vi "test number array to sgl array.vi"(10 "send values":string[](array[string])=["2", "19", "924", "0"]) -> (2 "sgl array":dbl[](array[numeric]))   [LabVIEW 2020]
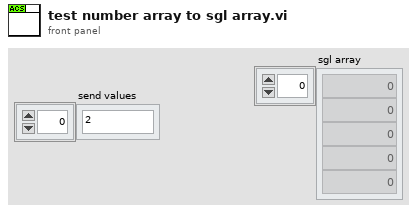
[diagram p1: front panel]
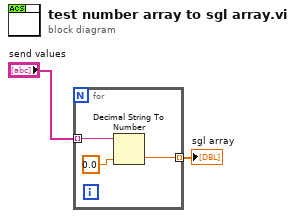
[diagram p0: block diagram]
diagram:
  n1 = for {
    tunnel: "send values" -> [w5] mode=indexing
    tunnel: [w3] -> w1 mode=indexing
    n2 = Decimal String To Number(string=w5, default (0L)=0.0) -> (number=w3:dbl)  [unwired: 1 in, 1 out]
  }
  "sgl array" <- w1
